vi "HGETALL.vi"(8 "error in (no error)":errorcluster, 10 "key":string, 11 "Redis Client in":refnum<class "Redis Client.lvclass">) -> (0 "error out":errorcluster, 2 "RESP3 Value":variant, 3 "Redis Client out":refnum<class "Redis Client.lvclass">)   [LabVIEW 2023, in "Redis Client for LabVIEW.lvlib" / "Redis Client.lvclass"]
uses:
  Redis Client.lvclass
  lib/RESP3-for-LabVIEW/RESP3/subVIs/RESP3 Make String Base.vi
  lib/RESP3-for-LabVIEW/RESP3/types/RESP3 data type attribute.vi
  lib/RESP3-for-LabVIEW/RESP3/RESP3.lvlib
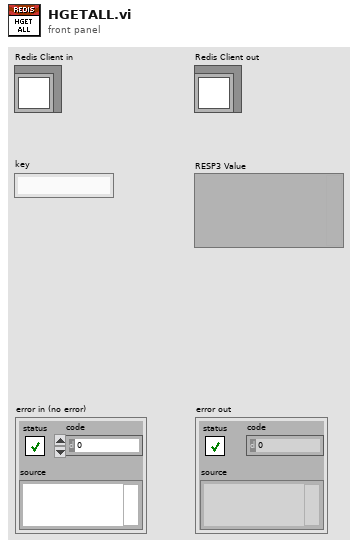
[diagram p1: front panel]
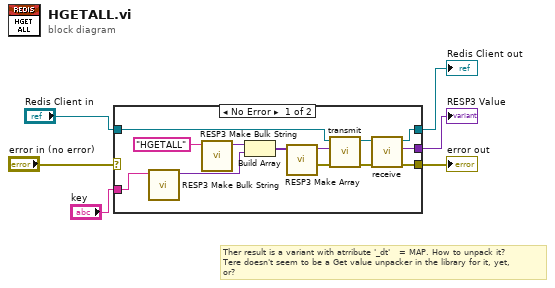
[diagram p0: block diagram]
diagram:
  # "Ther result is a variant with atrribute '_dt'   = MAP. How to unpack it?\nTere doesn't seem to be a Get value unpacker in the library for it, yet,\nor?"
  n1 = case shown="No Error" "error in (no error)" {
    selector: "error in (no error)" -> [_ w21]
    tunnel: [w10 w21] -> w5
    tunnel: "Redis Client in" -> [w19 w20]
    tunnel: [w12 w20] -> w3
    tunnel: "key" -> [w16 _]
    tunnel: [w11 _] -> w1
    frame No Error {
      n2 = call "RESP3 Make Bulk String.vi"("String"=w16) -> ("RESP3 Value out"=w15:variant)  [unwired: 9 in, 1 out]
      n3 = call "RESP3 Make Bulk String.vi"("String"="HGETALL" ("string in")) -> ("RESP3 Value out"=w14:variant)  [unwired: 9 in, 1 out]
      n4 = Build Array(w14, w15) -> (w18:variant[])
      n5 = call "RESP3 Make Array.vi"("RESP3 Values in"=w18) -> ("error out"=w8:errorcluster, "RESP3 Value out"=w7:variant)  [unwired: 9 in]
      n6 = call-dynamic "transmit.vi"("error in (no error)"=w8, "RESP3 Value"=w7, "Redis Client in"=w19) -> ("error out"=w9:errorcluster, "Redis Client out"=w13:refnum<class "Redis Client.lvclass">)  [unwired: 7 in]
      n7 = call-dynamic "receive.vi"("error in (no error)"=w9, "Redis Client in"=w13) -> ("error out"=w10:errorcluster, "RESP3 Value"=w11:variant, "Redis Client out"=w12:refnum<class "Redis Client.lvclass">)  [unwired: 6 in, 1 out]
    }
    frame Error {
    }
  }
  "error out" <- w5
  "Redis Client out" <- w3
  "RESP3 Value" <- w1
